vi "Interface_Dispatch_Process Module.vi"(8 "error in (no error)":errorcluster, 10 "TagBus DVR":refnum<data-value>, 11 "Dispatch_Demand Limiting in":refnum<class "Dispatch_Demand Limiting.lvclass">) -> (0 "error out":errorcluster, 2 "TagBus DVR out":refnum<data-value>, 3 "Dispatch_Demand Limiting out":refnum<class "Dispatch_Demand Limiting.lvclass">)   [LabVIEW 2015, in "Dispatch_Demand Limiting.lvclass"]
uses:
  Dispatch_Demand Limiting.lvclass
  TagBus/TagBus.lvclass
  Dispatch_Demand Limiting_Dependencies.ctl
  Dispatch_Demand Limiting_Configuration.ctl
  Dispatch_Demand Limiting_Output.ctl
panel:
  out "Output":T1
  in  "Configuration":T2
  in  "Dependencies":T3
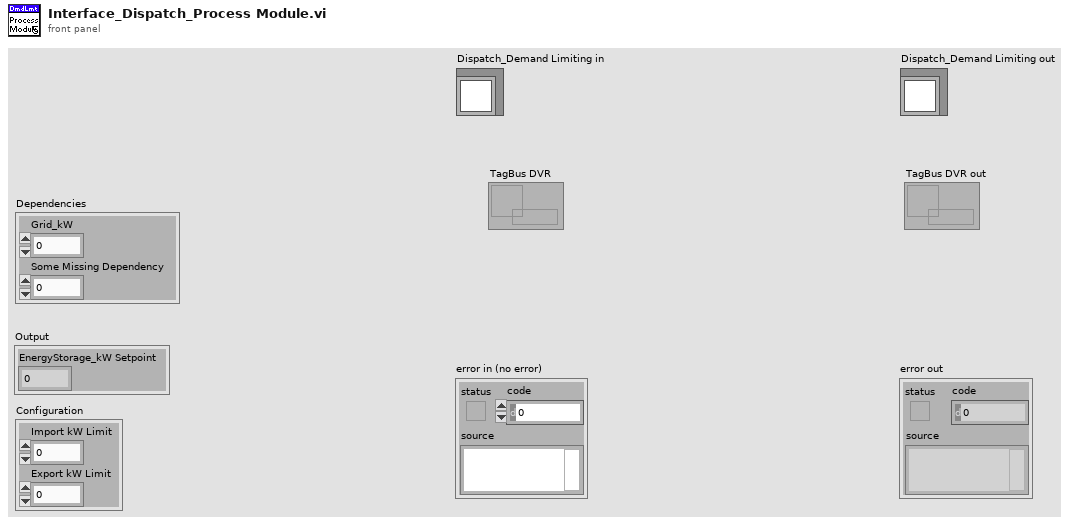
[diagram p1: front panel]
types:
  T1 = typedef "Dispatch_Demand Limiting.lvclass/Dispatch_Demand Limiting_Output.ctl" = cluster{"EnergyStorage_kW Setpoint":dbl}
  T2 = typedef "Dispatch_Demand Limiting.lvclass/Dispatch_Demand Limiting_Configuration.ctl" = cluster{"Import kW Limit":dbl, "Export kW Limit":dbl}
  T3 = typedef "Dispatch_Demand Limiting.lvclass/Dispatch_Demand Limiting_Dependencies.ctl" = cluster{"Grid_kW":dbl, "Some Missing Dependency":dbl}
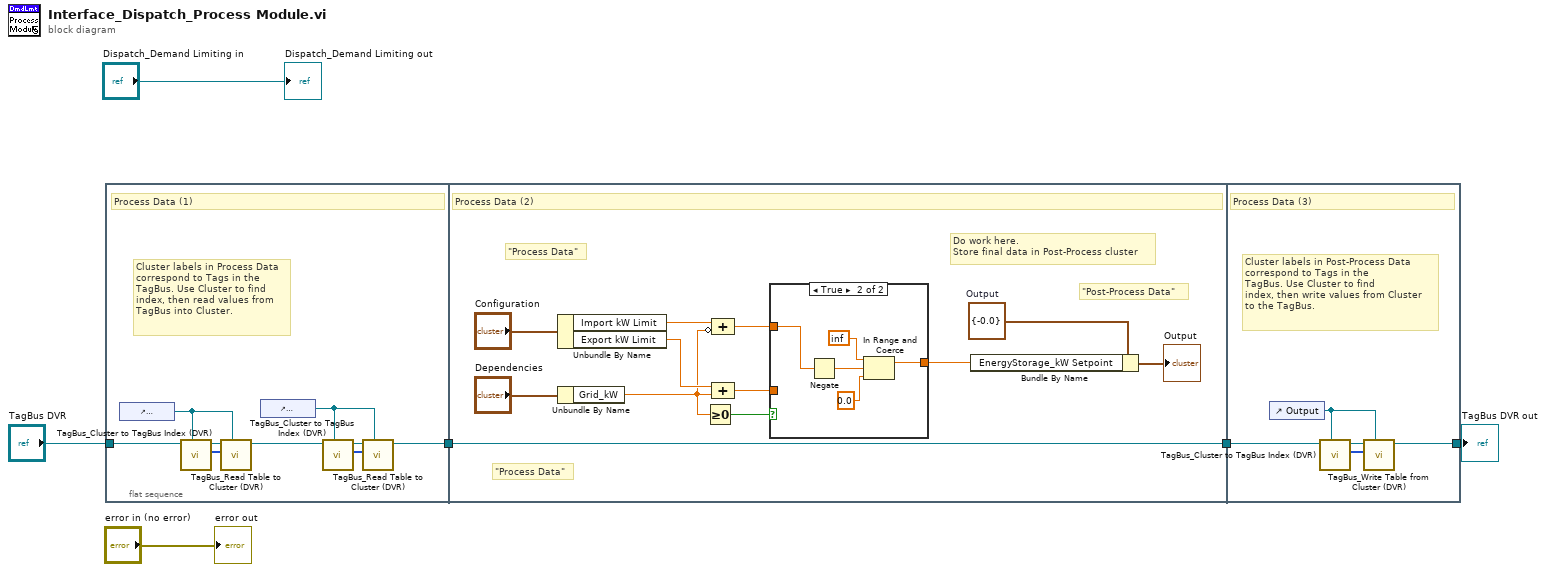
[diagram p0: block diagram]
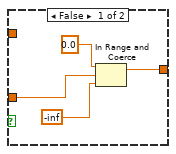
[diagram p2: hidden frame]
diagram:
  n1 = flat-sequence {
    tunnel: [w11] -> w6
    tunnel: "TagBus DVR" -> [w9]
    tunnel: w6 -> [w27]
    tunnel: [w27] -> w5
    tunnel: w5 -> [w41]
    tunnel: [w38] -> w2
    frame #0 {
      # "Cluster labels in Process Data\ncorrespond to Tags in the\nTagBus. Use Cluster to find\nindex, then read values from\nTagBus into Cluster."
      # "Process Data (1)"
      n2 = control-ref of="Configuration"() -> (w8:refnum<vi>)
      n3 = call "TagBus_Cluster to TagBus Index (DVR).vi"("Clust Refnum"=w8, "TagBus DVR"=w9) -> ("Index Array"=w15:i32[], "TagBus DVR out"=w14:refnum<data-value>)  [unwired: 8 in]
      n4 = call "TagBus_Read Table to Cluster (DVR).vi"("Clust Refnum"=w8, "Index Array"=w15, "TagBus DVR"=w14) -> ("TagBus DVR out"=w12:refnum<data-value>)  [unwired: 8 in]
      n5 = control-ref of="Dependencies"() -> (w7:refnum<vi>)
      n6 = call "TagBus_Cluster to TagBus Index (DVR).vi"("Clust Refnum"=w7, "TagBus DVR"=w12) -> ("Index Array"=w13:i32[], "TagBus DVR out"=w10:refnum<data-value>)  [unwired: 8 in]
      n7 = call "TagBus_Read Table to Cluster (DVR).vi"("Clust Refnum"=w7, "Index Array"=w13, "TagBus DVR"=w10) -> ("TagBus DVR out"=w11:refnum<data-value>)  [unwired: 8 in]
    }
    frame #1 {
      w26 = T1 {"EnergyStorage_kW Setpoint"=-0.0}  # Output
      # "\"Post-Process Data\""
      # "\"Process Data\""
      # "\"Process Data\""
      # "Do work here.\nStore final data in Post-Process cluster"
      # "Process Data (2)"
      n8 = Unbundle By Name("Configuration") -> ("Import kW Limit"=w22:dbl, "Export kW Limit"=w21:dbl)
      n9 = Unbundle By Name("Dependencies") -> ("Grid_kW"=w20:dbl)
      n10 = Greater Or Equal To 0?(x=w20) -> (x >= 0?=w19:bool)
      n11 = Compound Arithmetic op=ADD(w22, invert w20) -> (w17:dbl)
      n12 = Compound Arithmetic op=ADD(w21, w20) -> (w18:dbl)
      n13 = case shown="True" w19 {
        tunnel: w18 -> [w31 _]
        tunnel: w17 -> [_ w36]
        tunnel: [w28 w32] -> w16
        frame False {
          n14 = In Range and Coerce(upper limit=0.0, x=w31, lower limit=-inf) -> (coerced(x)=w28:dbl)  [unwired: 1 out]
        }
        frame True {
          n15 = Negate(x=w36) -> (-x=w35:dbl)
          n16 = In Range and Coerce(upper limit=inf, x=w35, lower limit=0.0) -> (coerced(x)=w32:dbl)  [unwired: 1 out]
        }
      }
      n17 = Bundle By Name(cluster=w26, "EnergyStorage_kW Setpoint"=w16) -> (→"Output":T1)
    }
    frame #2 {
      # "Cluster labels in Post-Process Data\ncorrespond to Tags in the\nTagBus. Use Cluster to find\nindex, then write values from Cluster\nto the TagBus."
      # "Process Data (3)"
      n18 = control-ref of="Output"() -> (w37:refnum<vi>)
      n19 = call "TagBus_Cluster to TagBus Index (DVR).vi"("Clust Refnum"=w37, "TagBus DVR"=w41) -> ("Index Array"=w40:i32[], "TagBus DVR out"=w39:refnum<data-value>)  [unwired: 8 in]
      n20 = call "TagBus_Write Table from Cluster (DVR).vi"("Clust Refnum"=w37, "Index Array"=w40, "Data Value Reference in"=w39) -> ("Data Value Reference out"=w38:refnum<data-value>)  [unwired: 8 in]
    }
  }
  "error out" <- "error in (no error)"
  "Dispatch_Demand Limiting out" <- "Dispatch_Demand Limiting in"
  "TagBus DVR out" <- w2
